vi "DataIn.vi"(8 "error in (no error)":errorcluster caption="错误输入（无错误）", 11 "XYPlot 输入":refnum<class "TrendPlot.lvclass">) -> (0 "error out":errorcluster caption="错误输出", 1 "Data1":dbl[](array[numeric]), 2 "Data0":dbl[](array[numeric]), 3 "XYPlot 输出":refnum<class "TrendPlot.lvclass">)   [LabVIEW 2018, in "DataDisplay.lvlib" / "TrendPlot.lvclass"]
uses:
  TrendPlot.lvclass
  TrendPlot.lvclass/TrendPlot.ctl
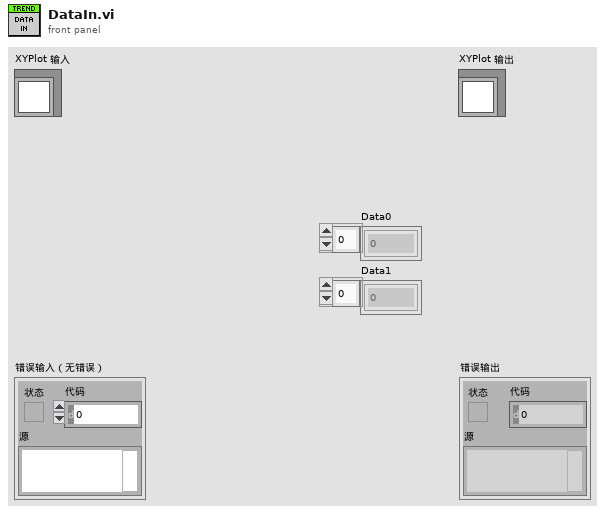
[diagram p1: front panel]
types:
  T1 = typedef "DataDisplay.lvlib/DD_DataStream.ctl" = cluster{"Data":dbl[]}[]
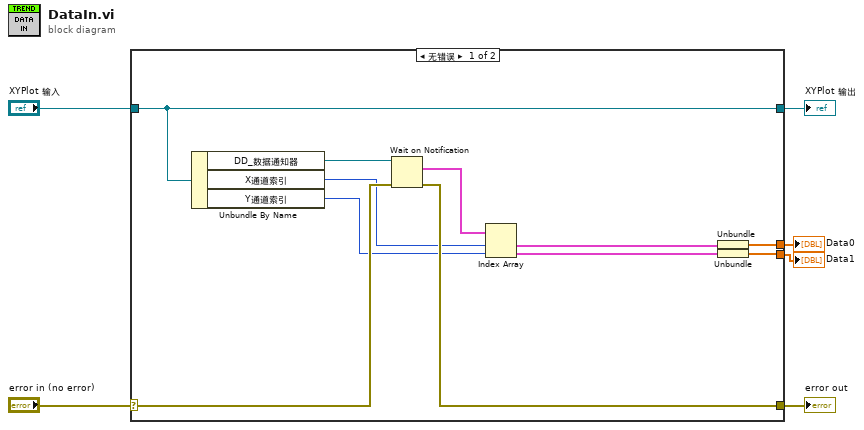
[diagram p0: block diagram]
diagram:
  n1 = case shown="无错误" "error in (no error)" {
    selector: "error in (no error)" -> [w14 w19]
    tunnel: [w13 w19] -> w5
    tunnel: [w17 w18] -> w3
    tunnel: "XYPlot 输入" -> [w17 w18]
    tunnel: [w10 _] -> w2
    tunnel: [w9 _] -> w1
    frame No Error {
      n2 = Unbundle By Name(w17) -> ("DD_数据通知器"=w15:refnum<notifier>, "X通道索引"=w12:i32, "Y通道索引"=w11:i32)
      n3 = Wait on Notification(notifier=w15, error in (no error)=w14) -> (notification=w16:T1, error out=w13:errorcluster)  [unwired: 2 in, 2 out]
      n4 = Index Array(array=w16, index #1=w12, index #2=w11) -> (element #1=w8:cluster{"Data":dbl[]}, element #2=w7:cluster{"Data":dbl[]})
      n5 = Unbundle(w8) -> ("Data"=w10:dbl[])
      n6 = Unbundle(w7) -> ("Data"=w9:dbl[])
    }
    frame Error {
    }
  }
  "error out" <- w5
  "XYPlot 输出" <- w3
  "Data0" <- w2
  "Data1" <- w1
